vi "数据查询_校准记录.vi"() -> ()   [LabVIEW 2016]
uses:
  <vilib>/Utility/miscctls.llb/LVRowAndColumnUnsignedTypeDef.ctl
  <vilib>/Utility/miscctls.llb/LVPointTypeDef.ctl
  <userlib>/_OpenG.lib/array/array.llb/Sort 2D Array (String)__ogtk.vi
panel:
  in  "下拉列表":string(xcontrol)
  in  "导出":bool
  in  "查询":bool
  in  "结束日期":string="2020/01/01"
  in  "起始日期":string="2010/01/01"
  in  "数据表":T1
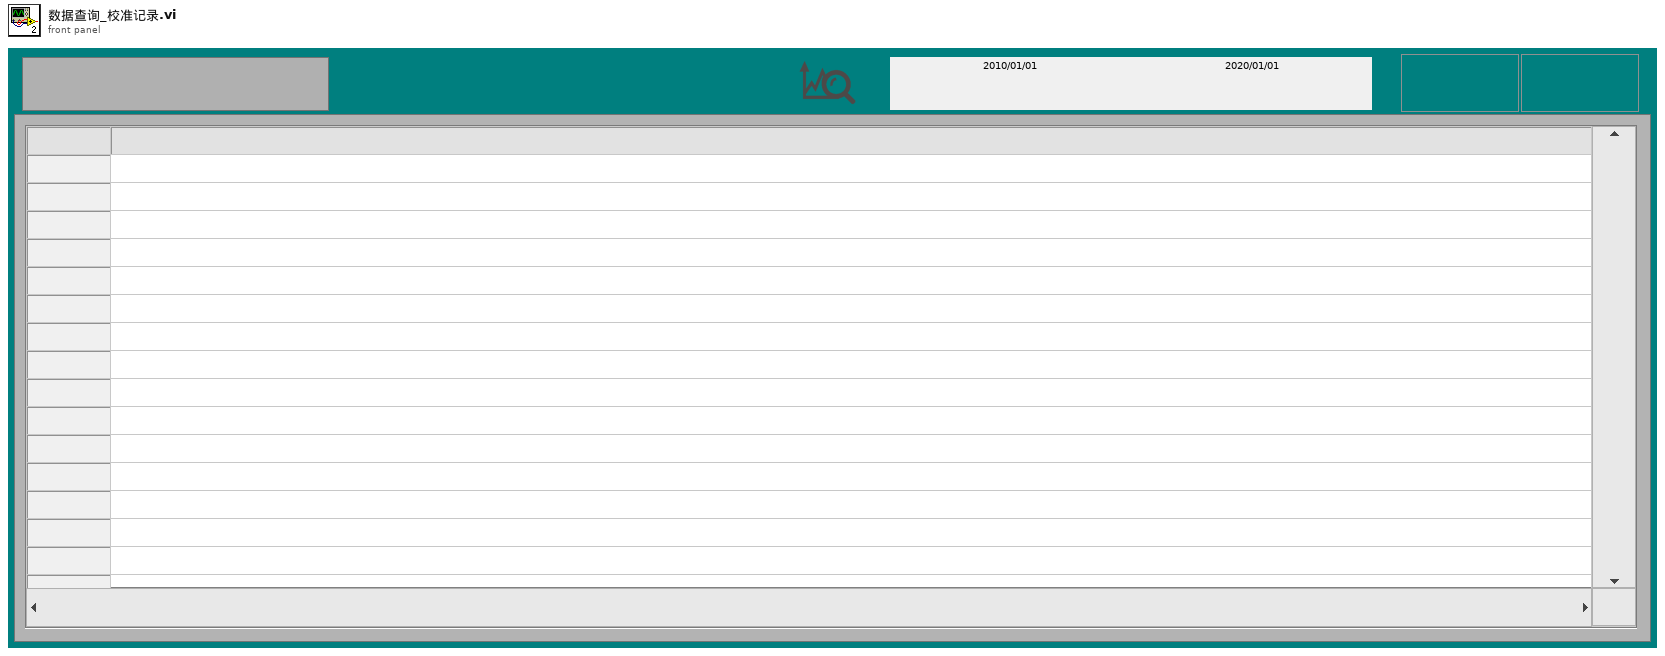
[diagram p1: front panel]
types:
  T1 = typedef "数据查询大列表框.ctl" = i32
  T2 = enum16{"Not Moving", "Mouse Down", "Douse Up", "Moving"}
  T3 = typedef "LVRowAndColumnUnsignedTypeDef.ctl" = cluster{"Row":u32, "Column":u32}
  T4 = typedef "LVPointTypeDef.ctl" = cluster{"Horizontal":i16, "Vertical":i16}
  T5 = cluster{"时间标识":timestamp, "设备":string, "日志信息":string, "流程参数":string}
  T6 = typedef "LVPoint32TypeDef.ctl" = cluster{"Horizontal":i32, "Vertical":i32}
  T7 = typedef "LVRowAndColumnTypeDef.ctl" = cluster{"Row":i32, "Column":i32}
  T8 = enum8{"Enabled", "Disabled", "Disabled and Grayed Out"}
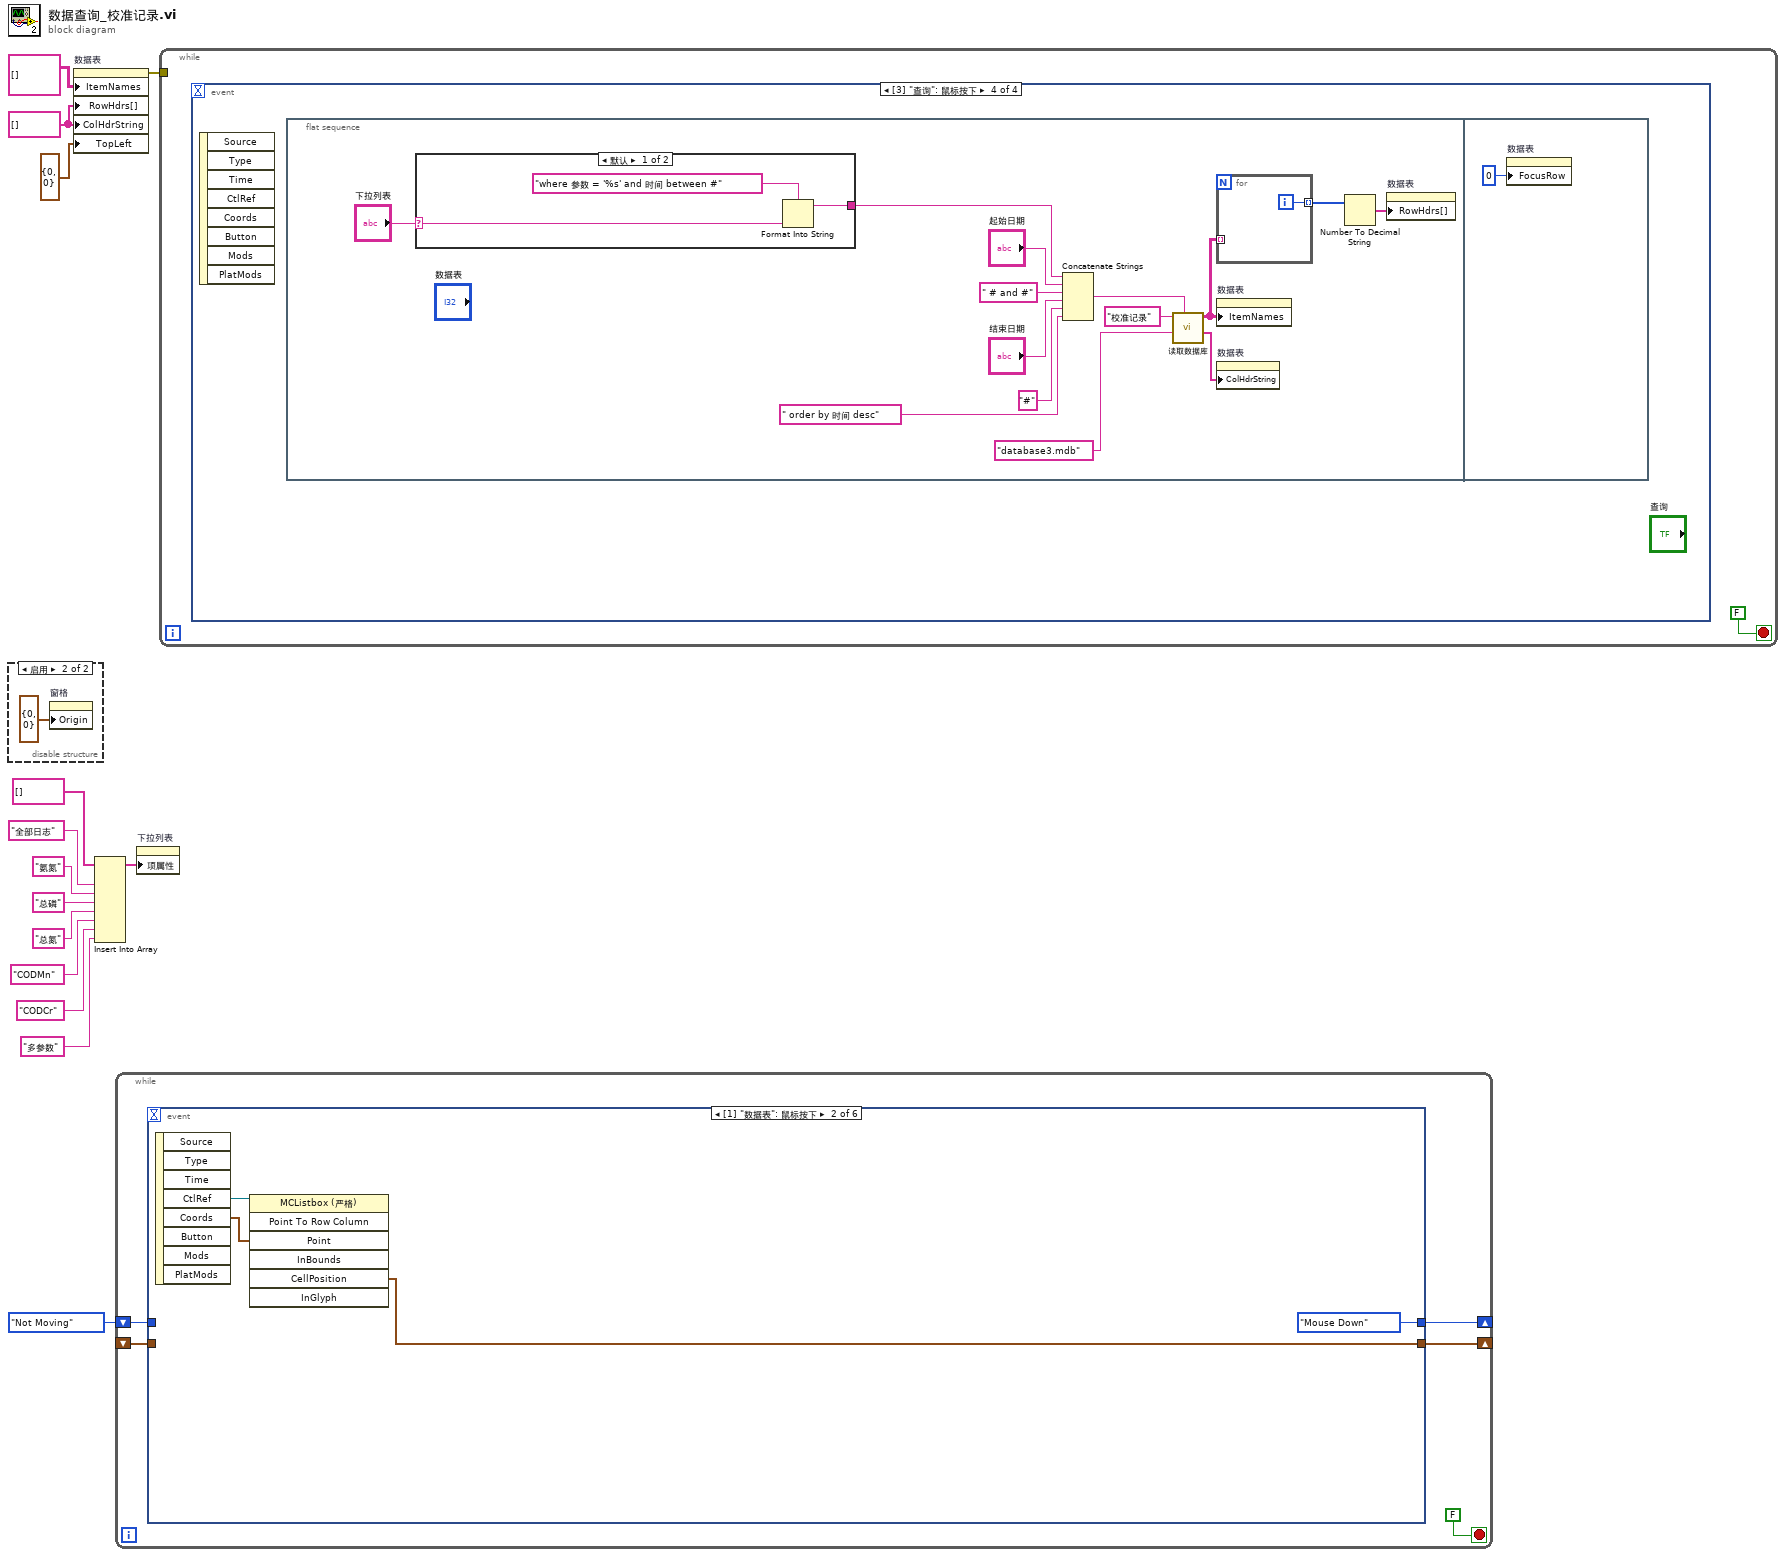
[diagram p0: block diagram]
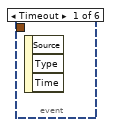
[diagram p2: hidden frame]
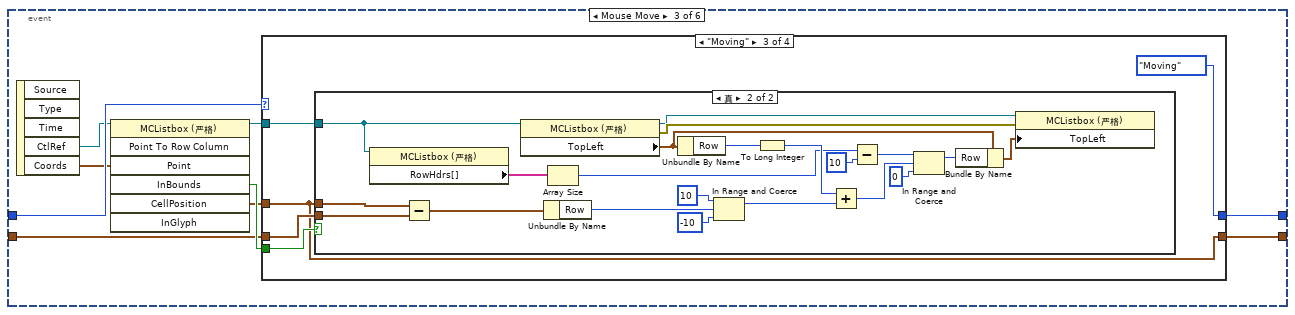
[diagram p3: hidden frame]
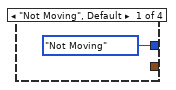
[diagram p4: hidden frame]
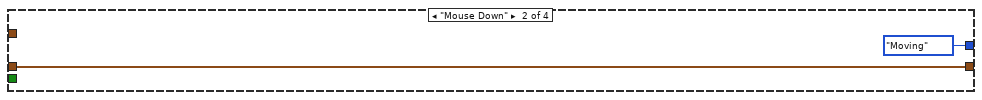
[diagram p5: hidden frame]
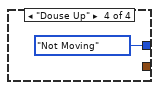
[diagram p7: hidden frame]
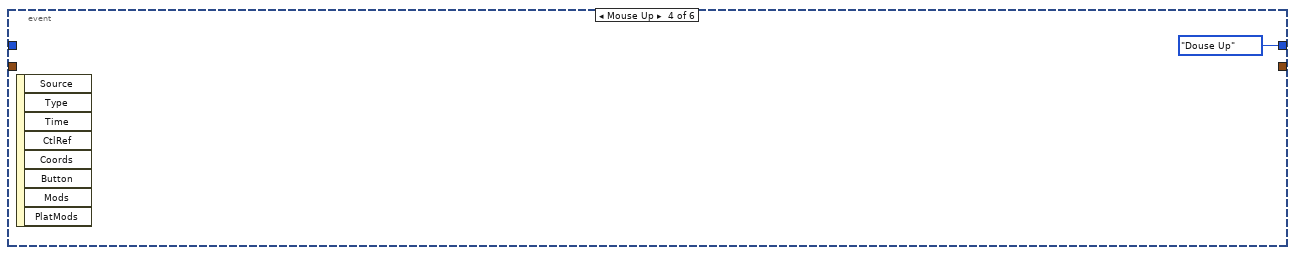
[diagram p8: hidden frame]
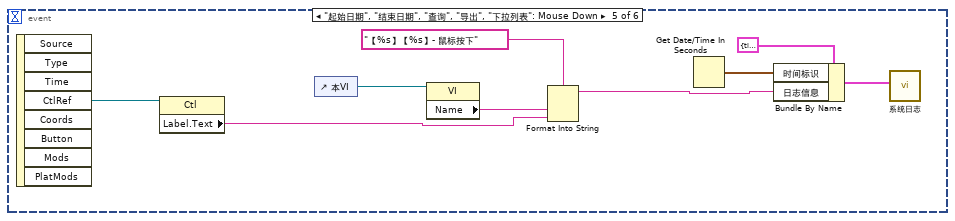
[diagram p9: hidden frame]
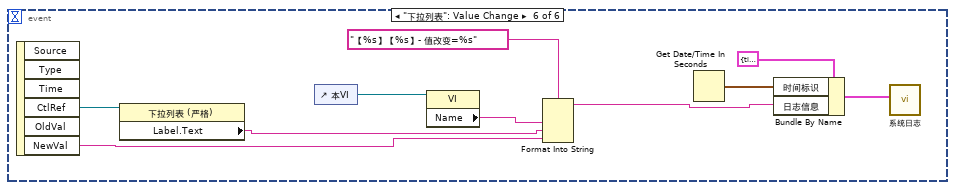
[diagram p10: hidden frame]
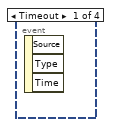
[diagram p11: hidden frame]
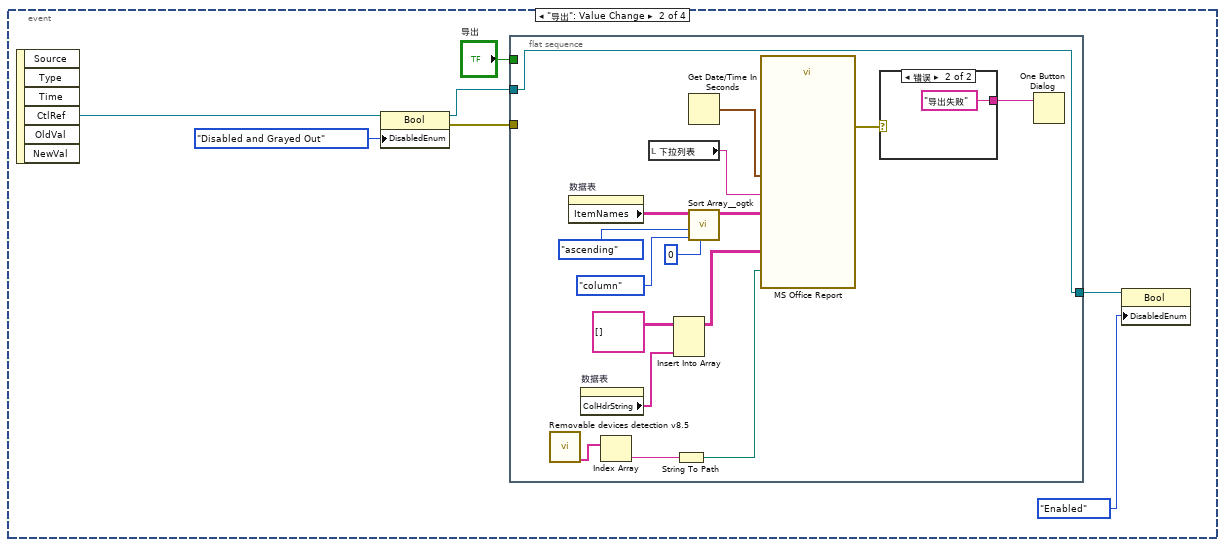
[diagram p12: hidden frame]
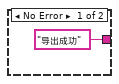
[diagram p13: hidden frame]
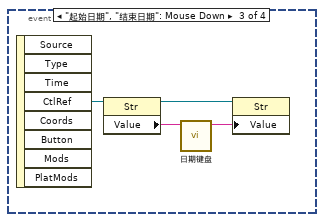
[diagram p14: hidden frame]
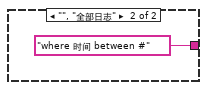
[diagram p15: hidden frame]
diagram:
  w3 = string[] [] ("行首字符串[]")
  n1 = disable-structure shown="启用" {
    frame Disabled {
    }
    frame Enabled {
      n2 = property on="窗格" class="Pane"("Origin"=T4 {"Horizontal"=0, "Vertical"=0} ("原点")) -> ()  [unwired: 2 in, 2 out]
    }
  }
  n3 = property on="数据表" class="MCListbox (严格)"("ItemNames"=string[][] [] ("项名"), "RowHdrs[]"=w3, "ColHdrString"=w3, "TopLeft"=T3 {"Row"=0, "Column"=0} ("左上可见单元格")) -> (error out=w5:errorcluster)  [unwired: 2 in, 1 out]
  n4 = Insert Into Array(array=string[] [], new element #1="全部日志" ("新元素/子数组"), new element #2="氨氮" ("新元素/子数组"), new element #3="总磷" ("新元素/子数组"), new element #4="总氮" ("新元素/子数组"), new element #5="CODMn" ("新元素/子数组"), new element #6="CODCr" ("新元素/子数组"), new element #7="多参数" ("新元素/子数组")) -> (w6:string[])  [unwired: 1 in]
  n5 = while {
    shift-right: [w18] -> _
    shift-left: T2."Not Moving" -> [w19]
    shift-right: [w17] -> _
    shift-left: _ -> [w16]
    stop <- FALSE stop-if-true
    n6 = event shown="[1] \"数据表\": 鼠标按下" {
      selector: _ -> [_ _ _ _ _ _]
      dyn-events: _ -> [_ _ _ _ _ _]
      timeout: _ -> [_ _ _ _ _ _]
      tunnel: w19 -> [_ _ w33 _ _ _]
      tunnel: [_ enum16{"Not Moving", "Mouse Down", "Douse Up"}."Mouse Down" w31 T2."Douse Up" _ _] -> w18
      tunnel: [_ w21 w32 _ _ _] -> w17
      tunnel: w16 -> [_ _ w26 _ _ _]
      event Timeout {
        n7 = event-data() -> ()  [unwired: 1 in, 3 out]
      }
      event Mouse Down {
        n8 = event-data() -> ("CtlRef"=w23:refnum<vi>, "Coords"=w22:T6)  [unwired: 1 in, 6 out]
        n9 = invoke class="MCListbox (严格)" method="Point To Row Column"(reference=w23, "Point"=w22) -> ("CellPosition"=w21:T7)  [unwired: 5 in, 6 out]
      }
      event Mouse Move {
        n10 = event-data() -> ("CtlRef"=w30:refnum<vi>, "Coords"=w29:T6)  [unwired: 1 in, 3 out]
        n11 = invoke class="MCListbox (严格)" method="Point To Row Column"(reference=w30, "Point"=w29) -> (reference out=w25:refnum<vi>, "InBounds"=w28:bool, "CellPosition"=w27:T7)  [unwired: 5 in, 4 out]
        n12 = case shown="\"Moving\"" w33 {
          tunnel: [_ w35 w38 _] -> w32
          tunnel: w26 -> [_ w35 w39 _]
          tunnel: [T2."Not Moving" T2."Moving" T2."Moving" T2."Not Moving"] -> w31
          tunnel: w28 -> [_ _ w40 _]
          tunnel: w27 -> [_ _ w38 _]
          tunnel: w25 -> [_ _ w37 _]
          frame "Not Moving", Default {
          }
          frame "Mouse Down" {
          }
          frame "Moving" {
            n13 = case shown="真" w40 {
              tunnel: w38 -> [_ w62]
              tunnel: w39 -> [_ w61]
              tunnel: w37 -> [_ w42]
              frame False {
              }
              frame True {
                n14 = property on="属性节点" class="MCListbox (严格)"(reference=w42) -> ("RowHdrs[]"=w53:string[])  [unwired: 1 in, 2 out]
                n15 = Subtract(x=w62, y=w61) -> (x-y=w57:T7)
                n16 = property on="属性节点" class="MCListbox (严格)"(reference=w42) -> (reference out=w43:refnum<vi>, error out=w60:errorcluster, "TopLeft"=w59:T3)  [unwired: 1 in]
                n17 = Unbundle By Name(w57) -> ("Row"=w50:i32)
                n18 = Array Size(array=w53) -> (size(s)=w45:i32)
                n19 = Unbundle By Name(w59) -> ("Row"=w52:u32)
                n20 = In Range and Coerce(upper limit=10 ("上限"), x=w50, lower limit=-10 ("下限")) -> (coerced(x)=w47:i32)  [unwired: 1 out]
                n21 = To Long Integer(number=w52) -> (32bit integer=w51:i32)
                n22 = Add(x=w51, y=w47) -> (x+y=w56:i32)
                n23 = Subtract(x=w45, y=10) -> (x-y=w46:i32)
                n24 = In Range and Coerce(upper limit=w46, x=w56, lower limit=0 ("下限")) -> (coerced(x)=w54:i32)  [unwired: 1 out]
                n25 = Bundle By Name(cluster=w59, "Row"=w54) -> (w58:T3)
                n26 = property on="属性节点" class="MCListbox (严格)"(reference=w43, error in=w60, "TopLeft"=w58) -> ()  [unwired: 2 out]
              }
            }
          }
          frame "Douse Up" {
          }
        }
      }
      event Mouse Up {
        n27 = event-data() -> ()  [unwired: 1 in, 8 out]
      }
      event "起始日期", "结束日期", "查询", "导出", "下拉列表": Mouse Down {
        n28 = event-data() -> ("CtlRef"=w70:refnum<vi>)  [unwired: 1 in, 7 out]
        n29 = property class="Ctl"(reference=w70) -> ("Label.Text"=w69:string)  [unwired: 1 in, 2 out]
        n30 = control-ref of="本VI"() -> (w73:refnum<vi>)
        n31 = property class="VI"(reference=w73) -> ("Name"=w72:string)  [unwired: 1 in, 2 out]
        n32 = Format Into String(format string="【%s】【%s】- 鼠标按下" ("格式字符串"), w72, w69) -> (resulting string=w66:string)  [unwired: 2 in, 1 out]
        n33 = Get Date/Time In Seconds() -> (seconds since 1Jan1904=w65:timestamp)
        n34 = Bundle By Name(cluster=T5 {"时间标识"=timestamp(0 s since 1904-01-01), "设备"="系统", "日志信息"="", "流程参数"=""} ("data in"), "时间标识"=w65, "日志信息"=w66) -> (w67:T5)
        n35 = call "系统日志.vi"("data in"=w67) -> ()  [unwired: 11 in]
      }
      event "下拉列表": Value Change {
        n36 = event-data() -> ("CtlRef"=w75:refnum<vi>, "NewVal"=w74:string)  [unwired: 1 in, 4 out]
        n37 = property class="下拉列表 (严格)"(reference=w75) -> ("Label.Text"=w80:string)  [unwired: 1 in, 2 out]
        n38 = control-ref of="本VI"() -> (w83:refnum<vi>)
        n39 = property class="VI"(reference=w83) -> ("Name"=w82:string)  [unwired: 1 in, 2 out]
        n40 = Format Into String(format string="【%s】【%s】- 值改变=%s" ("格式字符串"), w82, w80, w74) -> (resulting string=w77:string)  [unwired: 2 in, 1 out]
        n41 = Get Date/Time In Seconds() -> (seconds since 1Jan1904=w76:timestamp)
        n42 = Bundle By Name(cluster=T5 {"时间标识"=timestamp(0 s since 1904-01-01), "设备"="系统", "日志信息"="", "流程参数"=""} ("data in"), "时间标识"=w76, "日志信息"=w77) -> (w78:T5)
        n43 = call "系统日志.vi"("data in"=w78) -> ()  [unwired: 11 in]
      }
    }
  }
  n44 = property on="下拉列表" class="下拉列表 (严格)"("项属性"=w6) -> ()  [unwired: 2 in, 2 out]
  n45 = while {
    tunnel: w5 -> [_]
    stop <- FALSE stop-if-true
    n46 = event shown="[3] \"查询\": 鼠标按下" {
      selector: _ -> [_ _ _ _]
      dyn-events: _ -> [_ _ _ _]
      timeout: _ -> [_ _ _ _]
      event Timeout {
        n47 = event-data() -> ()  [unwired: 1 in, 3 out]
      }
      event "导出": Value Change {
        n48 = event-data() -> ("CtlRef"=w85:refnum<vi>)  [unwired: 1 in, 5 out]
        n49 = property class="Bool"(reference=w85, "DisabledEnum"=T8."Disabled and Grayed Out" ("禁用")) -> (reference out=w89:refnum<vi>, error out=w90:errorcluster)  [unwired: 1 in]
        n50 = flat-sequence {
          tunnel: w90 -> [_]
          tunnel: [w101] -> w88
          tunnel: w89 -> [w101]
          tunnel: "导出" -> [_]
          frame #0 {
            n51 = call "Removable devices detection v8.5.vi"() -> ("Removable"=w98:string[])  [unwired: 4 out]
            n52 = property on="数据表" class="MCListbox (严格)"() -> ("ItemNames"=w92:string[][])  [unwired: 2 in, 2 out]
            n53 = property on="数据表" class="MCListbox (严格)"() -> ("ColHdrString"=w94:string[])  [unwired: 2 in, 2 out]
            n54 = Index Array(array=w98) -> (element=w97:string)  [unwired: 1 in]
            n55 = local read "下拉列表"() -> (w102:string)
            n56 = Insert Into Array(array=string[][] [], new element=w94) -> (w93:string[][])  [unwired: 2 in]
            n57 = String To Path(string=w97) -> (path=w96:path)
            n58 = Get Date/Time In Seconds() -> (seconds since 1Jan1904=w107:timestamp)
            n59 = call-poly <userlib>:"Sort Array__ogtk.vi"("Column/Row to Sort By"=u32 0, "Sort By in"=enum16{"row", "column"}."column", "Order"=enum16{"ascending", "descending"}."ascending", "Array in"=w92) -> ("Sorted Array out"=w106:string[][])  [unwired: 4 in, 3 out]
            n60 = call "MS Office Report"("Path to Save Report"=w96, "导出日期"=w107, "监测参数"=w102, "数据输入"=w106, "字段定义"=w93) -> ("error out"=w100:errorcluster)  [unwired: 21 in, 1 out]
            n61 = case shown="错误" w100 {
              tunnel: ["导出成功" ("消息") "导出失败" ("消息")] -> w99
              frame No Error {
              }
              frame Error {
              }
            }
            n62 = One Button Dialog(message=w99) -> ()  [unwired: 1 in, 1 out]
          }
        }
        n63 = property class="Bool"(reference=w88, "DisabledEnum"=T8."Enabled" ("禁用")) -> ()  [unwired: 1 in, 2 out]
      }
      event "起始日期", "结束日期": Mouse Down {
        n64 = event-data() -> ("CtlRef"=w113:refnum<vi>)  [unwired: 1 in, 7 out]
        n65 = property class="Str"(reference=w113) -> (reference out=w111:refnum<vi>, "Value"=w112:string)  [unwired: 1 in, 1 out]
        n66 = call "日期键盘.vi"("原值"=w112) -> ("x+y"=w110:string)  [unwired: 10 in]
        n67 = property class="Str"(reference=w111, "Value"=w110) -> ()  [unwired: 1 in, 2 out]
      }
      event "查询": Mouse Down {
        n68 = event-data() -> ()  [unwired: 1 in, 8 out]
        n69 = flat-sequence {
          frame #0 {
            n70 = case shown="默认" "下拉列表" {
              selector: "下拉列表" -> [w128 _]
              tunnel: [w130 "where 时间 between #" ("condition")] -> w117
              frame Default {
                n71 = Format Into String(format string="where 参数 = '%s' and 时间 between #" ("condition"), w128) -> (resulting string=w130:string)  [unwired: 2 in, 1 out]
              }
              frame "", "全部日志" {
              }
            }
            n72 = Concatenate Strings(w117, "起始日期", " # and #" ("condition"), "结束日期", "#" ("condition"), " order by 时间 desc" ("字符串")) -> (w126:string)
            n73 = call "读取数据库.vi"("condition"=w126, "database"="database3.mdb", "组合框"="校准记录" ("字符串")) -> ("columns"=w122:string[], "表格"=w114:string[][])  [unwired: 5 in, 2 out]
            n74 = for {
              tunnel: w114 -> [_] mode=indexing
              tunnel: [w132] -> w120 mode=indexing
              i -> [w132]
            }
            n75 = property on="数据表" class="MCListbox (严格)"("ItemNames"=w114) -> ()  [unwired: 2 in, 2 out]
            n76 = property on="数据表" class="MCListbox (严格)"("ColHdrString"=w122) -> ()  [unwired: 2 in, 2 out]
            n77 = Number To Decimal String(number=w120) -> (decimal integer string=w119:string[])  [unwired: 1 in]
            n78 = property on="数据表" class="MCListbox (严格)"("RowHdrs[]"=w119) -> ()  [unwired: 2 in, 2 out]
          }
          frame #1 {
            n79 = property on="数据表" class="MCListbox (严格)"("FocusRow"=0 ("选中行")) -> ()  [unwired: 2 in, 2 out]
          }
        }
      }
    }
  }
